vi "Single Class_Multiple_State.vi"(4 "System_Delay(s)":dbl=0.01 min=0.0 max=86400.0 format="%#_13p", 5 "Time Target (s)":dbl=30.0 format="%#_13g", 6 "State_Interval_Time(s)":dbl=0.001 min=0.0 max=86400.0 format="%#_13p", 7 "State#":i32=1000) -> ()   [LabVIEW 2021]
uses:
  C:/Program Files (x86)/Hyper State Machine Framework/SSW_Hyper_State_Machine.lvlibp/State_Machine_Class/Main_State_Machine/Hyper_State_Machine.lvclass
  C:/Program Files (x86)/Hyper State Machine Framework/SSW_Hyper_State_Machine.lvlibp/State_Machine_Class/State_Machine_Module.llb/State Machine[].ctl
  C:/Program Files (x86)/Hyper State Machine Framework/SSW_Hyper_State_Machine.lvlibp/State_Machine_Class/State_Machine_Module.llb/Iterval.ctl
  C:/Program Files (x86)/Hyper State Machine Framework/SSW_Hyper_State_Machine.lvlibp/State_Machine_Class/State_Machine_Module.llb/Lock_Unlock.ctl
  C:/Program Files (x86)/Hyper State Machine Framework/SSW_Hyper_State_Machine.lvlibp
panel:
  out "Current State":string
  out "Show_Stop_Button":bool=TRUE
  in  "Unlock":bool
  in  "Reset":bool
  in  "Lock Even":bool
  in  "Lock Odd":bool
  in  "lock All":bool
  in  "Stop":bool
  out "Timing":dbl[](array[numeric])
  out "Lock":bool[](array[boolean])
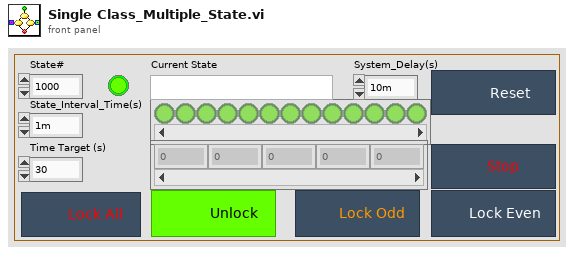
[diagram p1: front panel]
types:
  T1 = typedef "SSW_Hyper_State_Machine.lvlibp/State Machine.ctl" = cluster{"Command":string, "Data":variant}
  T2 = typedef "SSW_Hyper_State_Machine.lvlibp/State Machine[].ctl" = cluster{"Command":string, "Data":variant}[]
  T3 = typedef "SSW_Hyper_State_Machine.lvlibp/Lock_Unlock.ctl" = cluster{"Action_Mode (Get)":enum16{"Set", "Get"}, "Action_Set (False)":bool, "State_In (Wait)":string}
  T4 = typedef "SSW_Hyper_State_Machine.lvlibp/Iterval.ctl" = cluster{"Delay(s)":dbl, "State (Interval_Delay)":string}
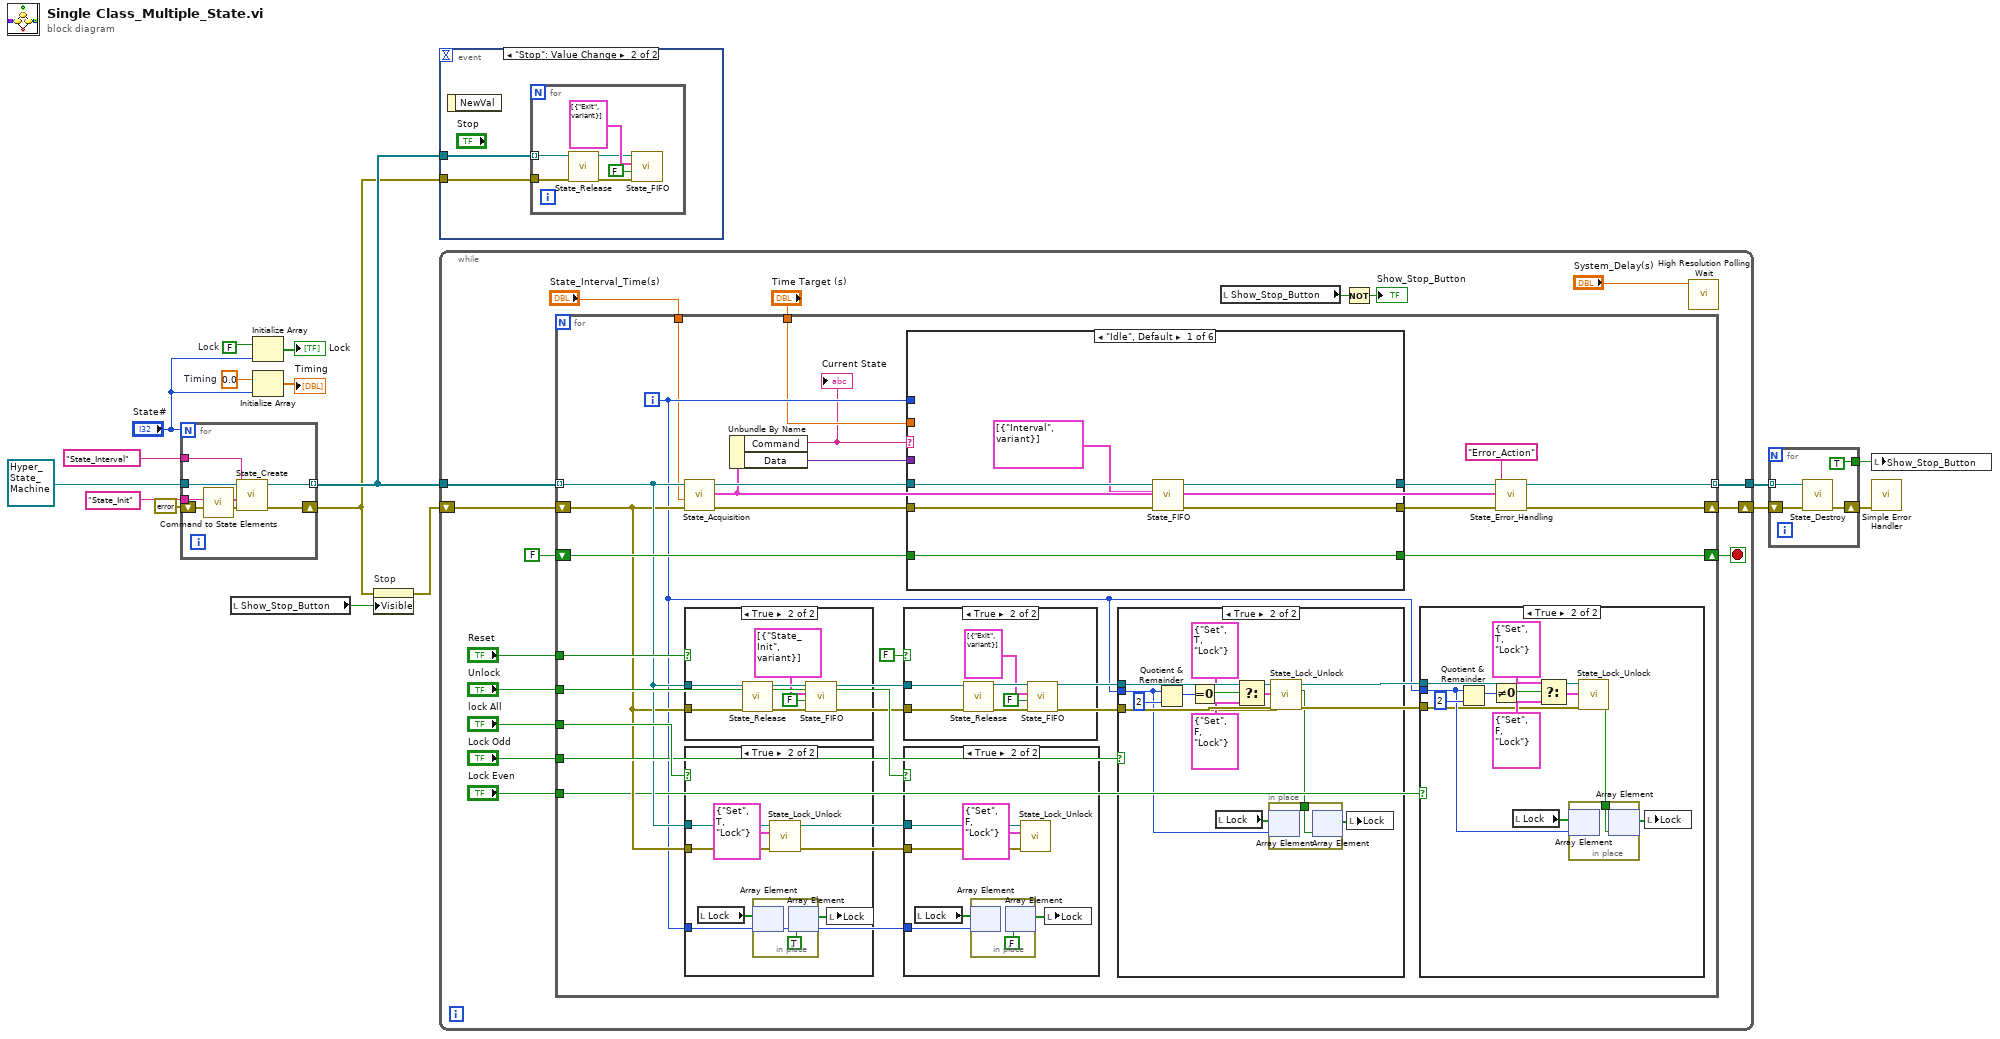
[diagram p0: block diagram]
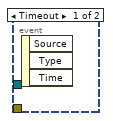
[diagram p2: hidden frame]
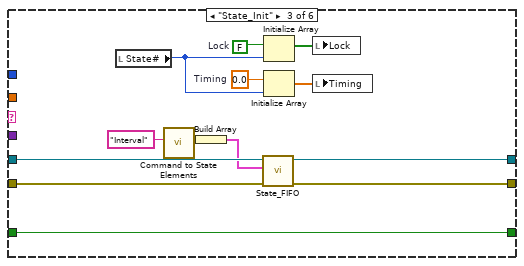
[diagram p10: hidden frame]
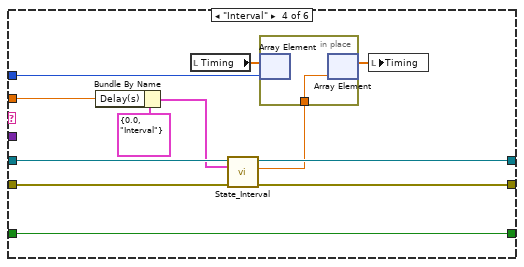
[diagram p11: hidden frame]
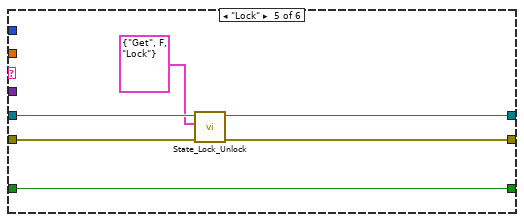
[diagram p12: hidden frame]
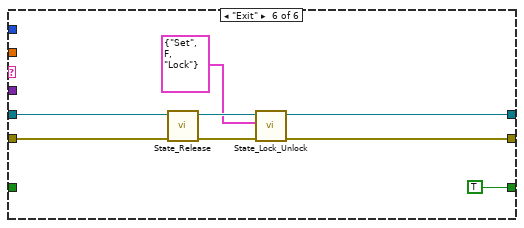
[diagram p13: hidden frame]
diagram:
  w11 = 0.0  # Timing
  w14 = FALSE  # Lock
  n1 = for {
    N: "State#" -> [_]
    tunnel: refnum<class "Hyper_State_Machine.lvclass"> refnum ("SSW_Hyper_State_Machine.lvlibp:Hyper_State_Machine.lvclass") -> [w24]
    tunnel: "State_Init" ("Command") -> [w22]
    tunnel: "State_Interval" ("Core_Interval_Name(State_Interval)") -> [w21]
    shift-right: [w20] -> w1
    shift-left: errorcluster {"status"=FALSE, "code"=0, "source"=""} ("error out") -> [w19]
    tunnel: [w18] -> w2 mode=indexing
    n2 = call "Command to State Elements.vi"("Command"=w22) -> ("Command to State Elements"=w23:T1)  [unwired: 10 in]
    n3 = call-dynamic "State_Create.vi"("error in (no error)"=w19, "Init_State(Option)"=w23, "State_Interval_Name"=w21, "State_Machine_Class in"=w24) -> ("error out"=w20:errorcluster, "State_Machine_Class out"=w18:refnum<class "Hyper_State_Machine.lvclass">)  [unwired: 5 in, 1 out]
  }
  n4 = local read "Show_Stop_Button"() -> (w4:bool)
  n5 = Initialize Array(w14, "State#") -> (→"Lock":bool[])
  n6 = Initialize Array(w11, "State#") -> (→"Timing":dbl[])
  n7 = property on="Stop" class="Bool"(error in=w1, "Visible"=w4) -> (error out=w5:errorcluster)  [unwired: 1 in, 1 out]
  n8 = event shown="[1] \"Stop\": Value Change" {
    selector: _ -> [_ _]
    dyn-events: _ -> [_ _]
    timeout: _ -> [_ _]
    tunnel: w2 -> [_ w26]
    tunnel: w1 -> [_ w25]
    event Timeout {
      n9 = event-data() -> ()  [unwired: 1 in, 3 out]
    }
    event "Stop": Value Change {
      n10 = event-data() -> ()  [unwired: 1 in, 1 out]
      n11 = for {
        tunnel: w26 -> [w28] mode=indexing
        tunnel: w25 -> [w27]
        n12 = call-dynamic "State_Release.vi"("error in (no error)"=w27, "State_Machine_Class in"=w28) -> ("error out"=w30:errorcluster, "State_Machine_Class out"=w29:refnum<class "Hyper_State_Machine.lvclass">)  [unwired: 8 in]
        n13 = call-dynamic "State_FIFO.vi"("error in (no error)"=w30, "State_Interval(Enable)"=FALSE, "State Machine[]"=T2 [{"Command"="Exit", "Data"=variant}], "State_Machine_Class in"=w29) -> ()  [unwired: 6 in, 2 out]
      }
    }
  }
  n14 = while {
    tunnel: w2 -> [w48]
    tunnel: [w44] -> w7
    shift-right: [w43] -> w6
    shift-left: w5 -> [w47]
    stop <- w46 stop-if-true
    n15 = for {
      tunnel: w48 -> [w56] mode=indexing
      shift-right: [w68] -> w43
      shift-left: w47 -> [w55]
      shift-right: [w63] -> w46
      shift-left: FALSE -> [w62]
      tunnel: [w61] -> w44 mode=indexing
      tunnel: "Reset" -> [w60]
      tunnel: "lock All" -> [w59]
      tunnel: "Unlock" -> [w58]
      tunnel: "Lock Odd" -> [w57]
      tunnel: "Lock Even" -> [w54]
      tunnel: "Time Target (s)" -> [w52]
      tunnel: "State_Interval_Time(s)" -> [w51]
      i -> [w53]
      n16 = call-dynamic "State_Acquisition.vi"("error in (no error)"=w55, "State_Interval_Time(s)"=w51, "Main_Machine_State_Class in"=w56) -> ("error out"=w69:errorcluster, "State"=w67:T1, "Main_Machine_State_Class out"=w70:refnum<class "Hyper_State_Machine.lvclass">)  [unwired: 2 in, 4 out]
      n17 = case shown="True" w60 {
        tunnel: w56 -> [_ w123]
        tunnel: w55 -> [_ w119]
        frame False {
        }
        frame True {
          n18 = call-dynamic "State_Release.vi"("error in (no error)"=w119, "State_Machine_Class in"=w123) -> ("error out"=w121:errorcluster, "State_Machine_Class out"=w122:refnum<class "Hyper_State_Machine.lvclass">)  [unwired: 8 in]
          n19 = call-dynamic "State_FIFO.vi"("error in (no error)"=w121, "State_Interval(Enable)"=FALSE, "State Machine[]"=T2 [{"Command"="State_Init", "Data"=variant}], "State_Machine_Class in"=w122) -> ()  [unwired: 6 in, 2 out]
        }
      }
      n20 = case shown="True" w59 {
        tunnel: w56 -> [_ w110]
        tunnel: w55 -> [_ w109]
        tunnel: w53 -> [_ w105]
        frame False {
        }
        frame True {
          n21 = local read "Lock"() -> (w107:bool[])
          n22 = in-place {
            n23 = in-place-array #1(w107, w105) -> ()  [unwired: 1 out]
            n24 = in-place-array #1(TRUE ("element")) -> (w106:bool[])  [unwired: 1 out]
          }
          n25 = call-dynamic "State_Lock_Unlock.vi"("error in (no error)"=w109, "Parameter"=T3 {"Action_Mode (Get)"=enum."Set", "Action_Set (False)"=TRUE, "State_In (Wait)"="Lock"}, "State_Machine_Class in"=w110) -> ()  [unwired: 6 in, 3 out]
          n26 = local write "Lock"(w106) -> ()
        }
      }
      n27 = Unbundle By Name(w67) -> ("Command"=w49:string, "Data"=w71:variant)
      "Current State" <- w49
      n28 = case shown="True" FALSE {
        tunnel: w56 -> [_ w117]
        tunnel: w55 -> [_ w113]
        frame False {
        }
        frame True {
          n29 = call-dynamic "State_Release.vi"("error in (no error)"=w113, "State_Machine_Class in"=w117) -> ("error out"=w115:errorcluster, "State_Machine_Class out"=w116:refnum<class "Hyper_State_Machine.lvclass">)  [unwired: 8 in]
          n30 = call-dynamic "State_FIFO.vi"("error in (no error)"=w115, "State_Interval(Enable)"=FALSE, "State Machine[]"=T2 [{"Command"="Exit", "Data"=variant}], "State_Machine_Class in"=w116) -> ()  [unwired: 6 in, 2 out]
        }
      }
      n31 = case shown="True" w58 {
        tunnel: w56 -> [_ w102]
        tunnel: w55 -> [_ w103]
        tunnel: w53 -> [_ w98]
        frame False {
        }
        frame True {
          n32 = local read "Lock"() -> (w99:bool[])
          n33 = in-place {
            n34 = in-place-array #2(w99, w98) -> ()  [unwired: 1 out]
            n35 = in-place-array #2(FALSE ("element")) -> (w100:bool[])  [unwired: 1 out]
          }
          n36 = call-dynamic "State_Lock_Unlock.vi"("error in (no error)"=w103, "Parameter"=T3 {"Action_Mode (Get)"=enum."Set", "Action_Set (False)"=FALSE, "State_In (Wait)"="Lock"}, "State_Machine_Class in"=w102) -> ()  [unwired: 6 in, 3 out]
          n37 = local write "Lock"(w100) -> ()
        }
      }
      n38 = case shown="\"Idle\", Default" w49 {
        tunnel: w71 -> [_ _ _ _ _ _]
        tunnel: w70 -> [w128 w132 w144 w151 w164 w171]
        tunnel: w69 -> [w127 w131 w142 w150 w163 w170]
        tunnel: [w126 w132 w143 w148 w162 w167] -> w65
        tunnel: [w125 w131 w141 w147 w161 w166] -> w64
        tunnel: w53 -> [_ _ _ w157 _ _]
        tunnel: [w129 w130 w145 w154 w159 TRUE] -> w63
        tunnel: w62 -> [w129 w130 w145 w154 w159 _]
        tunnel: w52 -> [_ _ _ w153 _ _]
        frame "Idle", Default {
          n39 = call-dynamic "State_FIFO.vi"("error in (no error)"=w127, "State Machine[]"=T2 [{"Command"="Interval", "Data"=variant}], "State_Machine_Class in"=w128) -> ("error out"=w125:errorcluster, "State_Machine_Class out"=w126:refnum<class "Hyper_State_Machine.lvclass">)  [unwired: 7 in]
        }
        frame "State_Interval" {
          # "Execute Every Define of State Interval Time"
        }
        frame "State_Init" {
          w137 = 0.0  # Timing
          w136 = FALSE  # Lock
          n40 = local read "State#"() -> (w135:i32)
          n41 = call "Command to State Elements.vi"("Command"="Interval") -> ("Command to State Elements"=w139:T1)  [unwired: 10 in]
          n42 = Build Array(w139) -> (w138:T1[])
          n43 = call-dynamic "State_FIFO.vi"("error in (no error)"=w142, "State Machine[]"=w138, "State_Machine_Class in"=w144) -> ("error out"=w141:errorcluster, "State_Machine_Class out"=w143:refnum<class "Hyper_State_Machine.lvclass">)  [unwired: 7 in]
          n44 = Initialize Array(w136, w135) -> (w133:bool[])
          n45 = Initialize Array(w137, w135) -> (w134:dbl[])
          n46 = local write "Lock"(w133) -> ()
          n47 = local write "Timing"(w134) -> ()
        }
        frame "Interval" {
          n48 = Bundle By Name(cluster=T4 {"Delay(s)"=0.0, "State (Interval_Delay)"="Interval"} ("Parameter"), "Delay(s)"=w153) -> (w149:T4)
          n49 = local read "Timing"() -> (w156:dbl[])
          n50 = call-dynamic "State_Interval.vi"("error in (no error)"=w150, "Parameter"=w149, "State_Machine_Class in"=w151) -> ("error out"=w147:errorcluster, "Elapsed Time(s)"=w146:dbl, "State_Machine_Class out"=w148:refnum<class "Hyper_State_Machine.lvclass">)  [unwired: 6 in]
          n51 = in-place {
            in-place-border: w146 -> [w158]
            n52 = in-place-array #3(w156, w157) -> ()  [unwired: 1 out]
            n53 = in-place-array #3(w158) -> (w155:dbl[])  [unwired: 1 out]
          }
          n54 = local write "Timing"(w155) -> ()
        }
        frame "Lock" {
          n55 = call-dynamic "State_Lock_Unlock.vi"("error in (no error)"=w163, "Parameter"=T3 {"Action_Mode (Get)"=enum."Get", "Action_Set (False)"=FALSE, "State_In (Wait)"="Lock"}, "State_Machine_Class in"=w164) -> ("error out"=w161:errorcluster, "State_Machine_Class out"=w162:refnum<class "Hyper_State_Machine.lvclass">)  [unwired: 6 in, 1 out]
        }
        frame "Exit" {
          n56 = call-dynamic "State_Release.vi"("error in (no error)"=w170, "State_Machine_Class in"=w171) -> ("error out"=w168:errorcluster, "State_Machine_Class out"=w169:refnum<class "Hyper_State_Machine.lvclass">)  [unwired: 8 in]
          n57 = call-dynamic "State_Lock_Unlock.vi"("error in (no error)"=w168, "Parameter"=T3 {"Action_Mode (Get)"=enum."Set", "Action_Set (False)"=FALSE, "State_In (Wait)"="Lock"}, "State_Machine_Class in"=w169) -> ("error out"=w166:errorcluster, "State_Machine_Class out"=w167:refnum<class "Hyper_State_Machine.lvclass">)  [unwired: 6 in, 1 out]
        }
      }
      n58 = case shown="True" w57 {
        tunnel: w53 -> [_ w88]
        tunnel: w56 -> [_ w86]
        tunnel: w55 -> [_ w85]
        frame False {
        }
        frame True {
          n59 = Quotient & Remainder(x=w88, y=2) -> (x-y*floor(x/y)=w95:i32)  [unwired: 1 out]
          n60 = Equal To 0?(x=w95) -> (x = 0?=w94:bool)
          n61 = local read "Lock"() -> (w90:bool[])
          n62 = Select(t=T3 {"Action_Mode (Get)"=enum."Set", "Action_Set (False)"=TRUE, "State_In (Wait)"="Lock"} ("Parameter"), s=w94, f=T3 {"Action_Mode (Get)"=enum."Set", "Action_Set (False)"=FALSE, "State_In (Wait)"="Lock"} ("Parameter")) -> (s? t:f=w91:T3)
          n63 = call-dynamic "State_Lock_Unlock.vi"("error in (no error)"=w85, "Parameter"=w91, "State_Machine_Class in"=w86) -> ("Action_Get"=w87:bool)  [unwired: 6 in, 2 out]
          n64 = in-place {
            in-place-border: w87 -> [w97]
            n65 = in-place-array #4(w90, w88) -> ()  [unwired: 1 out]
            n66 = in-place-array #4(w97) -> (w89:bool[])  [unwired: 1 out]
          }
          n67 = local write "Lock"(w89) -> ()
        }
      }
      n68 = case shown="True" w54 {
        tunnel: w53 -> [_ w75]
        tunnel: w56 -> [_ w73]
        tunnel: w55 -> [_ w72]
        frame False {
        }
        frame True {
          n69 = Quotient & Remainder(x=w75, y=2) -> (x-y*floor(x/y)=w82:i32)  [unwired: 1 out]
          n70 = Not Equal To 0?(x=w82) -> (x != 0?=w81:bool)
          n71 = local read "Lock"() -> (w77:bool[])
          n72 = Select(t=T3 {"Action_Mode (Get)"=enum."Set", "Action_Set (False)"=TRUE, "State_In (Wait)"="Lock"} ("Parameter"), s=w81, f=T3 {"Action_Mode (Get)"=enum."Set", "Action_Set (False)"=FALSE, "State_In (Wait)"="Lock"} ("Parameter")) -> (s? t:f=w78:T3)
          n73 = call-dynamic "State_Lock_Unlock.vi"("error in (no error)"=w72, "Parameter"=w78, "State_Machine_Class in"=w73) -> ("Action_Get"=w74:bool)  [unwired: 6 in, 2 out]
          n74 = in-place {
            in-place-border: w74 -> [w84]
            n75 = in-place-array #5(w77, w75) -> ()  [unwired: 1 out]
            n76 = in-place-array #5(w84) -> (w76:bool[])  [unwired: 1 out]
          }
          n77 = local write "Lock"(w76) -> ()
        }
      }
      n78 = call-dynamic "State_Error_Handling.vi"("error in (no error)"=w64, "Reply_State_Name"="Error_Action", "Handling_State(State_Acquisition)"=w67, "State_Machine_Class in"=w65) -> ("error out"=w68:errorcluster, "State_Machine_Class out"=w61:refnum<class "Hyper_State_Machine.lvclass">)  [unwired: 6 in]
    }
    n79 = local read "Show_Stop_Button"() -> (w34:bool)
    n80 = Not(x=w34) -> (.not. x?=→"Show_Stop_Button":bool)
    n81 = call <vilib>:"High Resolution Polling Wait.vi"("seconds to wait"="System_Delay(s)") -> ()  [unwired: 10 in, 1 out]
  }
  n82 = for {
    shift-right: [w176] -> w9
    shift-left: w6 -> [w175]
    tunnel: w7 -> [w174] mode=indexing
    tunnel: [TRUE ("Show_Stop_Button")] -> w3
    n83 = call-dynamic "State_Destroy.vi"("error in (no error)"=w175, "State_Machine_Class in"=w174) -> ("error out"=w176:errorcluster)  [unwired: 8 in, 1 out]
  }
  n84 = local write "Show_Stop_Button"(w3) -> ()
  n85 = call <vilib>:"Simple Error Handler.vi"("error in (no error)"=w9) -> ()  [unwired: 4 in, 5 out]
